vi "Move to cursor.vi"(4 "error in":errorcluster, 5 "input main cluster":T1) -> (0 "error out":errorcluster, 1 "output main cluster":T1)   [LabVIEW 2010]
uses:
  Main_cluster.ctl
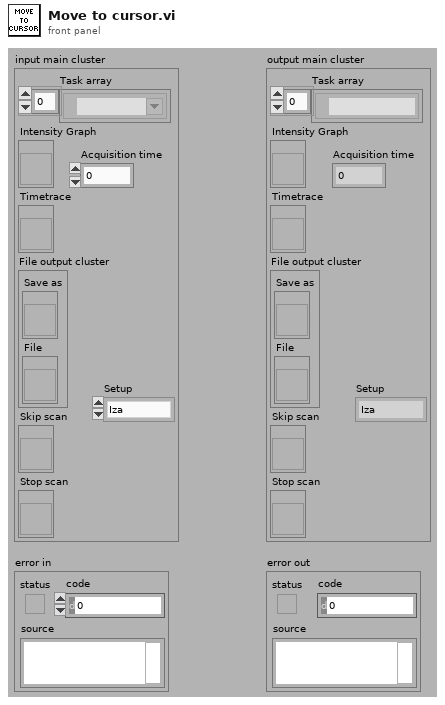
[diagram p1: front panel]
types:
  T1 = typedef "Main_cluster.ctl" = cluster{"Task array":refnum<k21>[], "Intensity Graph":refnum<vi>, "Timetrace":refnum<vi>, "File output cluster":cluster{"Save as":refnum<vi>, "File":refnum<vi>}, "Skip scan":refnum<vi>, "Stop scan":refnum<vi>, "Acquisition time":dbl, "Setup":enum16{"Iza", "Lukasz"}}
  T2 = typedef "LVPointDoubleTypeDef.ctl" = cluster{"Cursor X":dbl, "Cursor Y":dbl}
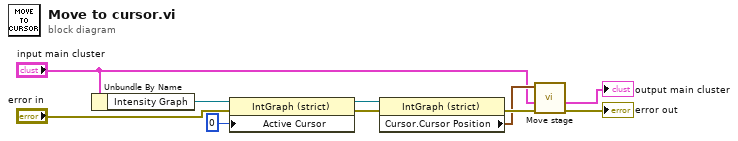
[diagram p0: block diagram]
diagram:
  n1 = Unbundle By Name("input main cluster") -> ("Intensity Graph"=w4:refnum<vi>)
  n2 = property on="Property Node" class="IntGraph (strict)"(reference=w4, error in="error in", "Active Cursor"=u32 0) -> (reference out=w3:refnum<vi>, error out=w6:errorcluster)
  n3 = property on="Property Node" class="IntGraph (strict)"(reference=w3, error in=w6) -> (error out=w8:errorcluster, "Cursor.Cursor Position"=w7:T2)  [unwired: 1 out]
  n4 = call "Move stage.vi"("error in"=w8, "input main cluster"="input main cluster", "Cursor.Cursor Position"=w7) -> ("error out"=→"error out":errorcluster, "output main cluster"=→"output main cluster":T1)  [unwired: 3 in]
